vi "oax_Cursor Handle.vi"(8 "error in (no error)":errorcluster, 11 "Order waveform":refnum<vi>) -> (0 "error out":errorcluster, 3 "Order waveform out":refnum<vi>)   [LabVIEW 2017]
panel:
  out "Cursor.Cursor X":dbl
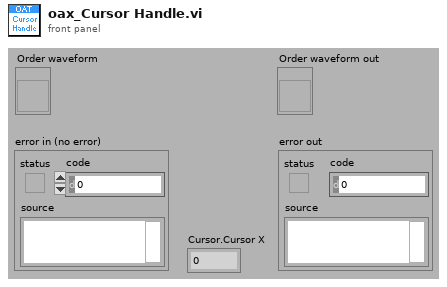
[diagram p1: front panel]
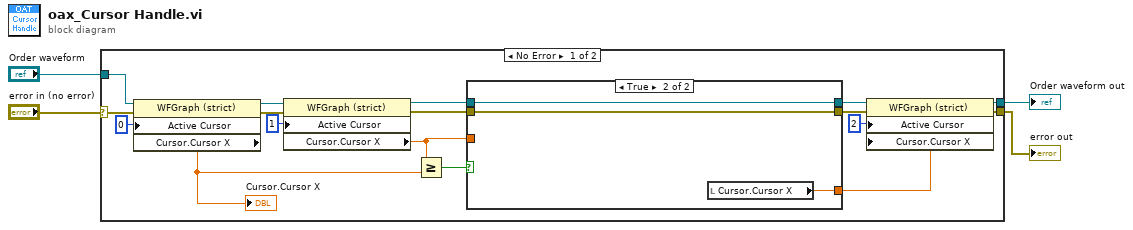
[diagram p0: block diagram]
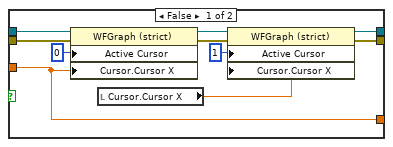
[diagram p2: hidden frame]
diagram:
  n1 = case shown="No Error" "error in (no error)" {
    selector: "error in (no error)" -> [w11 w35]
    tunnel: "Order waveform" -> [w21 w36]
    tunnel: [w9 w36] -> w3
    tunnel: [w7 w35] -> w2
    frame No Error {
      n2 = property class="WFGraph (strict)"(reference=w21, error in=w11, "Active Cursor"=u32 0) -> (reference out=w19:refnum<vi>, error out=w18:errorcluster, "Cursor.Cursor X"=w12:dbl)
      "Cursor.Cursor X" <- w12
      n3 = property class="WFGraph (strict)"(reference=w19, error in=w18, "Active Cursor"=u32 1) -> (reference out=w15:refnum<vi>, error out=w14:errorcluster, "Cursor.Cursor X"=w13:dbl)
      n4 = Greater Or Equal?(x=w13, y=w12) -> (x >= y?=w16:bool)
      n5 = case shown="True" w16 {
        tunnel: [w24 w34] -> w10
        tunnel: w15 -> [w31 w34]
        tunnel: [w23 w33] -> w8
        tunnel: w14 -> [w30 w33]
        tunnel: w13 -> [w22 _]
        tunnel: [w22 w32] -> w6
        frame False {
          n6 = property class="WFGraph (strict)"(reference=w31, error in=w30, "Active Cursor"=u32 0, "Cursor.Cursor X"=w22) -> (reference out=w28:refnum<vi>, error out=w27:errorcluster)
          n7 = local read "Cursor.Cursor X"() -> (w25:dbl)
          n8 = property class="WFGraph (strict)"(reference=w28, error in=w27, "Active Cursor"=u32 1, "Cursor.Cursor X"=w25) -> (reference out=w24:refnum<vi>, error out=w23:errorcluster)
        }
        frame True {
          n9 = local read "Cursor.Cursor X"() -> (w32:dbl)
        }
      }
      n10 = property class="WFGraph (strict)"(reference=w10, error in=w8, "Active Cursor"=u32 2, "Cursor.Cursor X"=w6) -> (reference out=w9:refnum<vi>, error out=w7:errorcluster)
    }
    frame Error {
    }
  }
  "Order waveform out" <- w3
  "error out" <- w2
